vi "Stop DQMH Module.vi"(8 "Module ID":i32, 9 "Module type":T1, 10 "Module Lib":refnum<vi>, 11 "References Map":map{string, refnum<vi>}(c390)) -> (0 "error out":errorcluster)   [LabVIEW 2019, in "Panther Dashboard.lvlib"]
uses:
  Panther Dashboard.lvlib
  Module type--enum.ctl
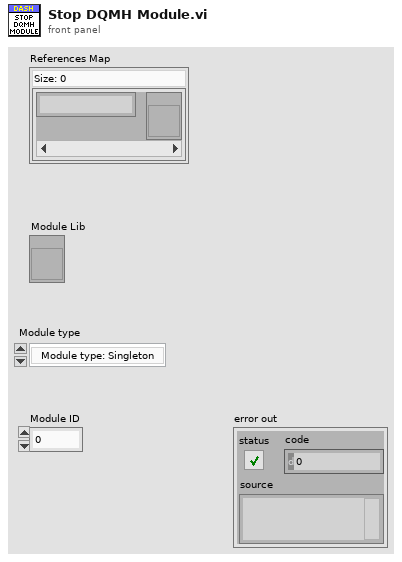
[diagram p1: front panel]
types:
  T1 = typedef "Panther Dashboard.lvlib/Module type--enum.ctl" = enum16{"Module type: Singleton", "Module type: Cloneable"}
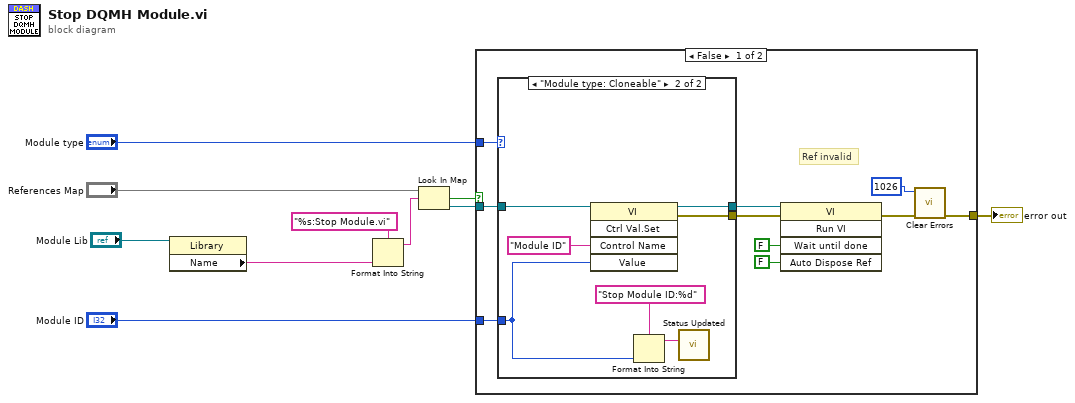
[diagram p0: block diagram]
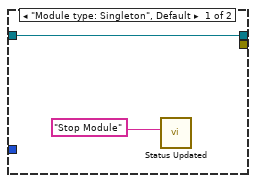
[diagram p2: hidden frame]
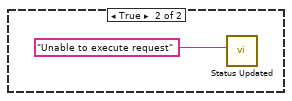
[diagram p3: hidden frame]
diagram:
  n1 = property class="Library"(reference="Module Lib") -> ("Name"=w3:string)  [unwired: 1 in, 2 out]
  n2 = Format Into String(format string="%s:Stop Module.vi", w3) -> (resulting string=w8:string)  [unwired: 2 in, 1 out]
  n3 = Look In Map(map="References Map", key=w8) -> (key not found?=w1:bool, value=w6:refnum<vi>)  [unwired: 1 in]
  n4 = case shown="False" w1 {
    tunnel: [w12 _] -> w10
    tunnel: w6 -> [w16 _]
    tunnel: "Module ID" -> [w15 _]
    tunnel: "Module type" -> [w13 _]
    frame False {
      # "Ref invalid"
      n5 = case shown="\"Module type: Cloneable\"" w13 {
        tunnel: [_ w29] -> w19
        tunnel: w16 -> [w22 w28]
        tunnel: w15 -> [_ w25]
        tunnel: [w22 w26] -> w14
        frame "Module type: Singleton", Default {
          n6 = call "Status Updated.vi"("Status"="Stop Module") -> ()  [unwired: 10 in, 1 out]
        }
        frame "Module type: Cloneable" {
          n7 = invoke class="VI" method="Ctrl Val.Set"(reference=w28, "Control Name"="Module ID", "Value"=w25) -> (reference out=w26:refnum<vi>, error out=w29:errorcluster)  [unwired: 2 in, 3 out]
          n8 = Format Into String(format string="Stop Module ID:%d" ("Status"), w25) -> (resulting string=w23:string)  [unwired: 2 in, 1 out]
          n9 = call "Status Updated.vi"("Status"=w23) -> ()  [unwired: 10 in, 1 out]
        }
      }
      n10 = invoke class="VI" method="Run VI"(reference=w14, error in=w19, "Wait until done"=FALSE ("Wait Until Done"), "Auto Dispose Ref"=FALSE ("Auto Dispose Reference")) -> (error out=w20:errorcluster)  [unwired: 1 in, 4 out]
      n11 = call <vilib>:"Clear Errors.vi"("error in (no error)"=w20, "specific error code to clear (0: all)"=1026) -> ("error out"=w12:errorcluster)  [unwired: 4 in, 1 out]
    }
    frame True {
      n12 = call "Status Updated.vi"("Status"="Unable to execute request") -> ()  [unwired: 10 in, 1 out]
    }
  }
  "error out" <- w10
